vi "EVM_5G_Freq_Sweep_Only.vi"() -> ()   [LabVIEW 2023, in "EVM.lvlib"]
uses:
  EVM.lvlib
  lib/Keysight/Keysight.lvlib
panel:
  out "SA Frequency(MHz)":i32
  out "SG Frequency(MHz)":i32
  out "SG Power":i32
  in  "SA_Freq(MHz)":i32[](array[numeric])
  in  "SG_Freq(MHz)":i32[](array[numeric])
  in  "Type":enum16{"Default", "E6680A"}(ring)
  in  "Waiting Time(ms)":u32=100
  in  "FileNote":string
  in  "Stop Power":i32=21
  in  "Start Power":i32=-20
  in  "SG":refnum<visa-resource-name>="TCPIP0::192.168.100.201::inst0::INSTR"
  in  "AvgTimes":i32=1
  in  "SA":refnum<visa-resource-name>="TCPIP0::192.168.100.202::inst0::INSTR"
  out "5G_EVM_Data":cluster{"X":dbl, "Y":dbl}[](graph)
  # "Keysigh 5G EVM \n             with Frequency Sweep"
  # "Setting"
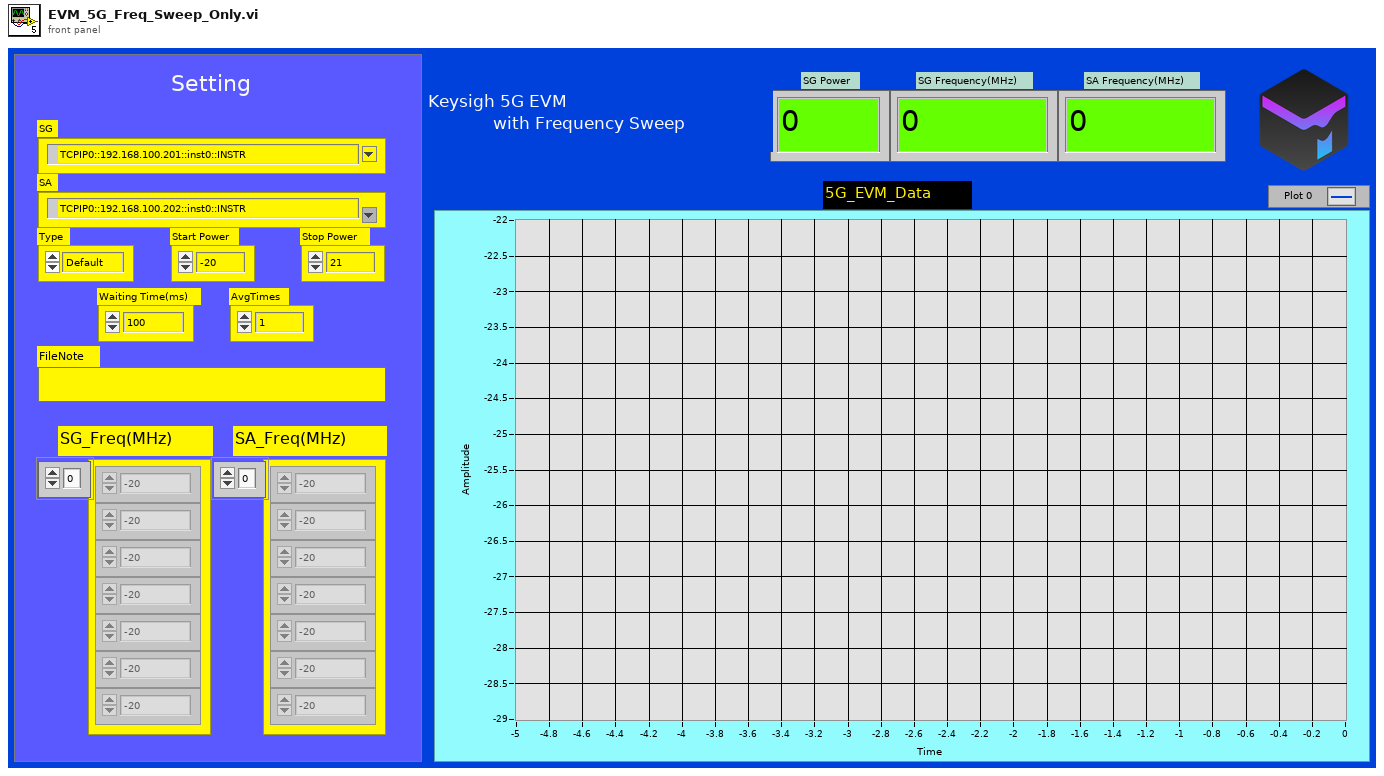
[diagram p1: front panel]
types:
  T1 = cluster{"Ch_POW_Total":dbl, "Ch_POW_Active":dbl, "EVM_RMS":dbl, "Freq_Error":dbl}
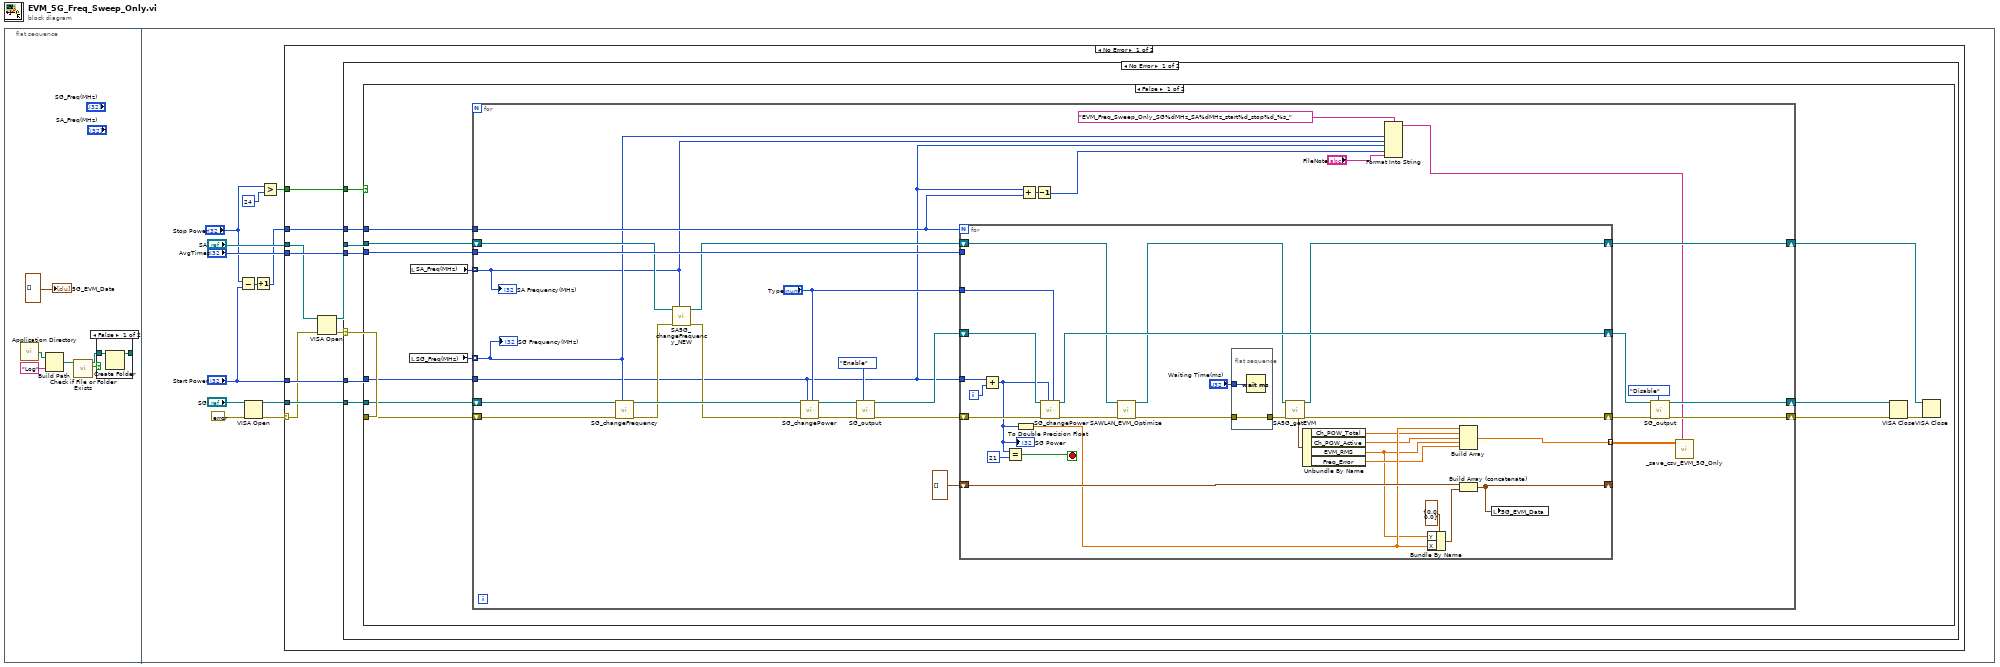
[diagram p0: block diagram]
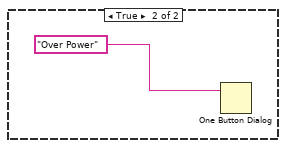
[diagram p3: hidden frame]
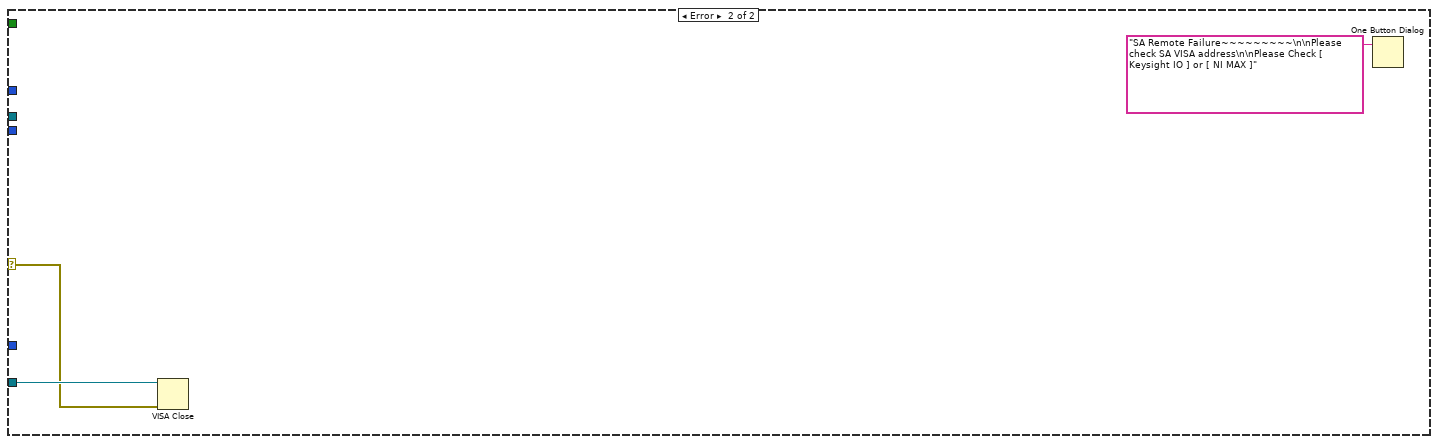
[diagram p4: hidden frame]
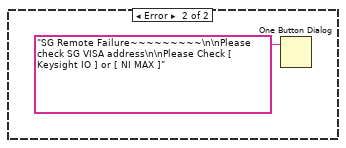
[diagram p5: hidden frame]
diagram:
  n1 = flat-sequence {
    frame #0 {
      n2 = call <vilib>:"Application Directory.vi"() -> ("Application Directory"=w5:path)
      n3 = Build Path(base path=w5, name or relative path="Log") -> (appended path=w2:path)
      n4 = call <vilib>:"Check if File or Folder Exists.vi"("path"=w2) -> ("file or folder exists?"=w4:bool, "dup path"=w3:path)  [unwired: 8 in, 1 out]
      n5 = case shown="False" w4 {
        tunnel: w3 -> [w8 w9]
        tunnel: [w7 w9] -> _
        frame False {
          n6 = Create Folder(path (use dialog)=w8) -> (created path=w7:path)  [unwired: 2 in, 2 out]
        }
        frame True {
        }
      }
      "5G_EVM_Data" <- cluster{"X":dbl, "Y":dbl}[] [] ("XY Graph")
    }
    frame #1 {
      n7 = Subtract(x="Stop Power", y="Start Power") -> (x-y=w17:i32)
      n8 = VISA Open(error in (no error)=errorcluster {"status"=FALSE, "code"=0, "source"=""}, VISA resource name="SG") -> (VISA resource name=w11:refnum<visa-resource-name>, error out=w10:errorcluster)  [unwired: 3 in]
      n9 = Increment(x=w17) -> (x+1=w16:i32)
      n10 = Greater?(x="Stop Power", y=24) -> (0:w20:bool)
      n11 = case shown="No Error" w10 {
        selector: w10 -> [w25 _]
        tunnel: "SA" -> [w23 _]
        tunnel: w20 -> [w30 _]
        tunnel: "Start Power" -> [w29 _]
        tunnel: "AvgTimes" -> [w28 _]
        tunnel: w16 -> [w27 _]
        tunnel: w11 -> [w26 _]
        frame No Error {
          n12 = VISA Open(error in (no error)=w25, VISA resource name=w23) -> (VISA resource name=w22:refnum<visa-resource-name>, error out=w24:errorcluster)  [unwired: 3 in]
          n13 = case shown="No Error" w24 {
            selector: w24 -> [w31 w112]
            tunnel: w22 -> [w37 _]
            tunnel: w30 -> [w36 _]
            tunnel: w29 -> [w35 _]
            tunnel: w28 -> [w34 _]
            tunnel: w27 -> [w33 _]
            tunnel: w26 -> [w32 w113]
            frame No Error {
              n14 = case shown="False" w36 {
                tunnel: w37 -> [w49 _]
                tunnel: w34 -> [w48 _]
                tunnel: w35 -> [w40 _]
                tunnel: w31 -> [w47 _]
                tunnel: w32 -> [w46 _]
                tunnel: w33 -> [w45 _]
                frame False {
                  n15 = local read "SG_Freq(MHz)"() -> (w39:i32[])
                  n16 = local read "SA_Freq(MHz)"() -> (w38:i32[])
                  n17 = for {
                    tunnel: w48 -> [w80]
                    tunnel: w45 -> [w74]
                    tunnel: w40 -> [w52]
                    shift-right: [w68] -> w41
                    shift-left: w49 -> [w60]
                    shift-right: [w70] -> w44
                    shift-left: w47 -> [w63]
                    shift-right: [w69] -> w43
                    shift-left: w46 -> [w62]
                    tunnel: w39 -> [w54] mode=indexing
                    tunnel: w38 -> [w53] mode=indexing
                    n18 = call "SG_changeFrequency.vi"("MHz"=w54, "error in"=w63, "VISA in"=w62) -> ("error out"=w58:errorcluster, "VISA out"=w61:refnum<visa-resource-name>)  [unwired: 6 in, 1 out]
                    n19 = call "SA5G_changeFrequency_NEW.vi"("MHz"=w53, "error in"=w58, "VISA in"=w60) -> ("error out"=w57:errorcluster, "VISA out"=w59:refnum<visa-resource-name>)  [unwired: 6 in, 1 out]
                    n20 = call "SG_changePower.vi"("Type"="Type", "dBm"=w52, "error in"=w57, "VISA in"=w61) -> ("error out"=w76:errorcluster, "VISA out"=w75:refnum<visa-resource-name>)  [unwired: 5 in, 1 out]
                    n21 = call "SG_output.vi"("Func."=enum16{"Disable", "Enable"}."Enable", "error in"=w76, "VISA in"=w75) -> ("error out"=w79:errorcluster, "VISA out"=w73:refnum<visa-resource-name>)  [unwired: 7 in]
                    n22 = for {
                      N: w74 -> [_]
                      tunnel: w80 -> [_]
                      tunnel: w52 -> [w106]
                      shift-right: [w101] -> w78
                      shift-left: w79 -> [w108]
                      shift-right: [w103] -> w72
                      shift-left: w73 -> [w102]
                      shift-right: [w98] -> w68
                      shift-left: w59 -> [w90]
                      shift-right: [w94] -> _
                      shift-left: cluster{"X":dbl, "Y":dbl}[] [] ("XY Graph") -> [w96]
                      tunnel: [w88] -> w66 mode=indexing
                      tunnel: "Type" -> [w86]
                      i -> [w107]
                      stop <- w104 stop-if-true
                      n23 = Add(x=w106, y=w107) -> (x+y=w93:i32)
                      "SG Power" <- w93
                      n24 = Equal?(x=w93, y=21) -> (x = y?=w104:bool)
                      n25 = To Double Precision Float(number=w93) -> (double precision float=w87:dbl)
                      n26 = call "SG_changePower.vi"("Type"=w86, "dBm"=w93, "error in"=w108, "VISA in"=w102) -> ("error out"=w92:errorcluster, "VISA out"=w103:refnum<visa-resource-name>)  [unwired: 5 in, 1 out]
                      n27 = call "SAWLAN_EVM_Optimize.vi"("error in"=w92, "VISA in"=w90) -> ("error out"=w91:errorcluster, "VISA out"=w89:refnum<visa-resource-name>)  [unwired: 8 in]
                      n28 = flat-sequence {
                        tunnel: w91 -> [w110]
                        tunnel: [w110] -> w100
                        tunnel: "Waiting Time(ms)" -> [w109]
                        frame #0 {
                          n29 = Wait (ms)(milliseconds to wait=w109) -> ()  [unwired: 1 out]
                        }
                      }
                      n30 = call "SA5G_getEVM.vi"("error in"=w100, "VISA in"=w89) -> ("error out"=w101:errorcluster, "VISA out"=w98:refnum<visa-resource-name>, "get_EVM"=w85:T1)  [unwired: 7 in]
                      n31 = Unbundle By Name(w85) -> ("Ch_POW_Total"=w82:dbl, "Ch_POW_Active"=w84:dbl, "EVM_RMS"=w81:dbl, "Freq_Error"=w83:dbl)
                      n32 = Bundle By Name(cluster=cluster{"X":dbl, "Y":dbl} {"X"=0.0, "Y"=0.0} ("element"), "Y"=w81, "X"=w87) -> (w95:cluster{"X":dbl, "Y":dbl})
                      n33 = Build Array(w87, w82, w84, w81, w83) -> (w88:dbl[])
                      n34 = Build Array (concatenate)(w96, w95) -> (w94:cluster{"X":dbl, "Y":dbl}[])
                      n35 = local write "5G_EVM_Data"(w94) -> ()
                    }
                    n36 = Add(x=w52, y=w74) -> (x+y=w77:i32)
                    n37 = Decrement(x=w77) -> (x-1=w51:i32)
                    n38 = Format Into String(format string="EVM_Freq_Sweep_Only_SG%dMHz_SA%dMHz_start%d_stop%d_%s_" ("delimiter (\\t)"), w54, w53, w52, w51, "FileNote") -> (resulting string=w55:string)  [unwired: 2 in, 1 out]
                    n39 = call "SG_output.vi"("Func."=enum16{"Disable", "Enable"}."Disable", "error in"=w78, "VISA in"=w72) -> ("error out"=w70:errorcluster, "VISA out"=w69:refnum<visa-resource-name>)  [unwired: 7 in]
                    n40 = call "_save_csv_EVM_5G_Only.vi"("delimiter (\\t)"=w55, "Data"=w66) -> ()  [unwired: 9 in, 1 out]
                    "SG Frequency(MHz)" <- w54
                    "SA Frequency(MHz)" <- w53
                  }
                  n41 = VISA Close(VISA resource name=w43, error in (no error)=w44) -> (error out=w42:errorcluster)
                  n42 = VISA Close(VISA resource name=w41, error in (no error)=w42) -> ()  [unwired: 1 out]
                }
                frame True {
                  n43 = One Button Dialog(message="Over Power") -> ()  [unwired: 1 in, 1 out]
                }
              }
            }
            frame Error {
              n44 = VISA Close(VISA resource name=w113, error in (no error)=w112) -> ()  [unwired: 1 out]
              n45 = One Button Dialog(message="SA Remote Failure~~~~~~~~~\n\nPlease check SA VISA address\n\nPlease Check [ Keysight IO ] or [ NI MAX ]") -> ()  [unwired: 1 in, 1 out]
            }
          }
        }
        frame Error {
          n46 = One Button Dialog(message="SG Remote Failure~~~~~~~~~\n\nPlease check SG VISA address\n\nPlease Check [ Keysight IO ] or [ NI MAX ]") -> ()  [unwired: 1 in, 1 out]
        }
      }
    }
  }
